vi "autoDrive.vi"(4 "Distance":dbl) -> (0 "right speed":dbl, 1 "left speed":dbl, 2 "finished?":bool)   [LabVIEW 2013]
doc: "Will drive the robot at a specified speed for a specified distance. Pretty simple."
uses:
  typedefs/fg_typedef.ctl
  typedefs/State Machine/subStates.ctl
  <vilib>/addons/control/pid/NI_PID_pid.lvlib
  <vilib>/addons/control/pid/pid.llb/PID (DBL).vi
panel:
  out "right desired rate":dbl
  out "left desired rate":dbl
  out "leftDistance":dbl
  out "rightDistance":dbl
  out "leftRate":dbl
  out "rightRate":dbl
  # "Encoder Data"
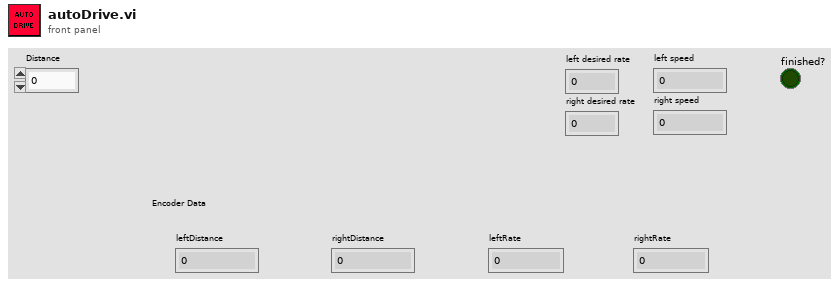
[diagram p1: front panel]
types:
  T1 = typedef "subStates.ctl" = enum16{"null", "wait", "driver control", "auto", "manual override", "hold position", "rotate", "pickup", "pass", "recover pass", "load", "goto shoot", "shoot high goal", "shoot low goal", "cancel arm", "cancel shooter", "end", "test"}
  T2 = typedef "fg_typedef.ctl" = enum16{"Get", "Set"}
  T3 = typedef "WPI_EncoderDevRef.ctl" = cluster{"DevStatus":errorcluster, "EncoderIndex":T4, "CounterIndex":T5, "DistancePerCount":dbl, "Decoding Type":T6}
  T4 = typedef "FPGA_EncoderIdx.ctl" = enum8{"Enc 0", "Enc 1", "Enc 2", "Enc 3", "Invalid"}
  T5 = typedef "FPGA_CounterCtrSystemIndex.ctl" = enum8{"Ctr 0", "Ctr 1", "Ctr 2", "Ctr 3", "Ctr 4", "Ctr 5", "Ctr 6", "Ctr 7", "Invalid"}
  T6 = typedef "WPI_EncoderType.ctl" = enum16{"1x", "2x", "4x"}
  T7 = cluster{"proportional gain (Kc)":dbl, "integral time (Ti, min)":dbl, "derivative time (Td, min)":dbl}
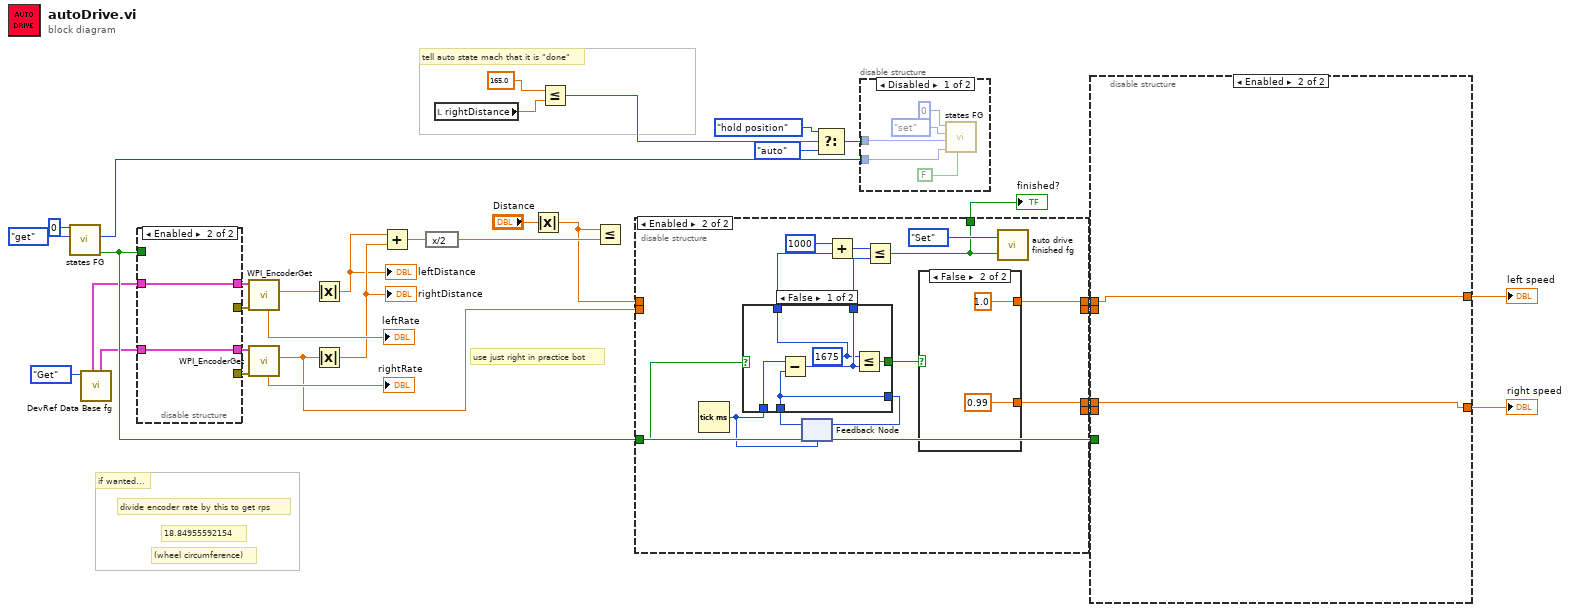
[diagram p0: block diagram]
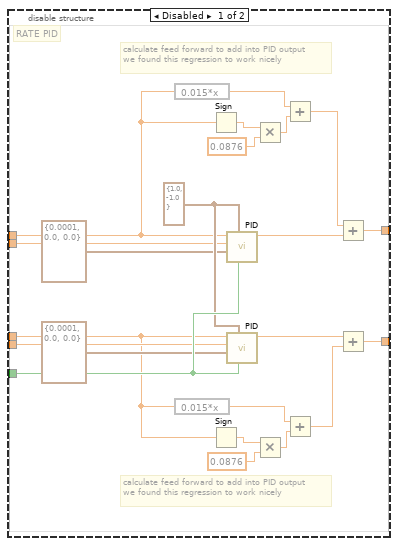
[diagram p3: hidden frame]
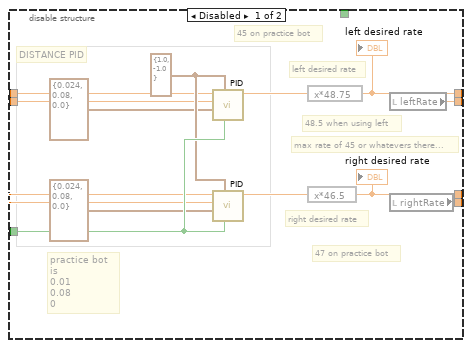
[diagram p4: hidden frame]
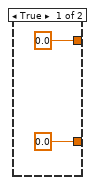
[diagram p5: hidden frame]
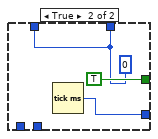
[diagram p6: hidden frame]
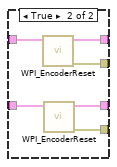
[diagram p8: hidden frame]
diagram:
  # "if wanted..."
  # "tell auto state mach that it is \"done\""
  # "use just right in practice bot"
  # "(wheel circumference)"
  # "divide encoder rate by this to get rps"
  # "18.84955592154"
  n1 = call "states FG.vi"("menu (get)"=enum16{"set", "get"}."get", "Loop ID"=0) -> ("first call?"=w34:bool, "state # out"=w26:i32)  [unwired: 6 in, 2 out]
  n2 = call "DevRef Data Base fg.vi"("Menu"=fg_typedef."Get") -> ("right drive encoder"=w23:T3, "left drive encoder"=w24:T3)  [unwired: 2 in, 7 out]
  n3 = disable-structure shown="Enabled" {
    disable-tunnel: w24 -> [w41 w51]
    disable-tunnel: w23 -> [w40 w50]
    disable-tunnel: [w39 _] -> w32
    disable-tunnel: [w38 w51] -> w31
    disable-tunnel: [w37 w50] -> w30
    disable-tunnel: [w36 _] -> w29
    disable-tunnel: w34 -> [w35 _]
    frame Disabled {
      n4 = case shown="False" w35 {
        tunnel: w41 -> [w43 w48]
        tunnel: w40 -> [w42 w46]
        tunnel: [_ w49] -> w39
        tunnel: [w43 w47] -> w38
        tunnel: [w42 w45] -> w37
        tunnel: [_ w44] -> w36
        frame False {
        }
        frame True {
          n5 = call <vilib>:"WPI_EncoderReset.vi"("EncoderDevRef"=w48) -> ("error out"=w49:errorcluster, "EncoderDevRef"=w47:T3)  [unwired: 9 in]
          n6 = call <vilib>:"WPI_EncoderReset.vi"("EncoderDevRef"=w46) -> ("error out"=w44:errorcluster, "EncoderDevRef"=w45:T3)  [unwired: 9 in]
        }
      }
    }
    frame Enabled {
    }
  }
  n7 = call <vilib>:"WPI_EncoderGet.vi"("error in (no error)"=w32, "EncoderDevRef"=w31) -> ("Distance"=w4:dbl, "Rate"=→"leftRate":dbl)  [unwired: 4 in, 4 out]
  n8 = call <vilib>:"WPI_EncoderGet.vi"("error in (no error)"=w29, "EncoderDevRef"=w30) -> ("Distance"=w3:dbl, "Rate"=→"rightRate":dbl)  [unwired: 4 in, 4 out]
  n9 = Absolute Value(x=w4) -> (abs(x)=w11:dbl)
  "leftDistance" <- w11
  n10 = Absolute Value(x=w3) -> (abs(x)=w14:dbl)
  "rightDistance" <- w14
  n11 = Add(x=w11, y=w14) -> (x+y=w13:dbl)
  n12 = expression code="x/2"(w13) -> (w12:dbl)
  n13 = local read "rightDistance"() -> (w8:dbl)
  n14 = Absolute Value(x="Distance") -> (abs(x)=w7:dbl)
  n15 = Less Or Equal?(x=165.0, y=w8) -> (x <= y?=w2:bool)
  n16 = Less Or Equal?(x=w7, y=w12) -> ()  [unwired: 1 out]
  n17 = disable-structure shown="Enabled" {
    disable-tunnel: w34 -> [w63 w71]
    disable-tunnel: [w58 _] -> w18
    disable-tunnel: [w57 _] -> w17
    disable-tunnel: [w56 w76] -> w16
    disable-tunnel: [w54 w75] -> w15
    disable-tunnel: w7 -> [w53 _]
    disable-tunnel: w3 -> [w52 _]
    disable-tunnel: [_ w67] -> w1
    frame Disabled {
      w60 = cluster{"output high":dbl, "output low":dbl} {"output high"=1.0, "output low"=-1.0} ("output range")
      # "DISTANCE PID"
      # "48.5 when using left"
      # "practice bot is \n0.01\n0.08\n0"
      # "45 on practice bot"
      # "47 on practice bot"
      # "max rate of 45 or whatevers there..."
      # "left desired rate"
      # "right desired rate"
      n18 = call-poly <vilib>:"PID.vi"("reinitialize? (F)"=w63, "output range"=w60, "PID gains"=T7 {"proportional gain (Kc)"=0.024, "integral time (Ti, min)"=0.08, "derivative time (Td, min)"=0.0} ("Left Distance PID gains"), "process variable"=w52, "setpoint"=w53) -> ("output"=w62:dbl)  [unwired: 5 in, 1 out]
      n19 = call-poly <vilib>:"PID.vi"("reinitialize? (F)"=w63, "output range"=w60, "PID gains"=T7 {"proportional gain (Kc)"=0.024, "integral time (Ti, min)"=0.08, "derivative time (Td, min)"=0.0} ("Right Distance PID gains"), "process variable"=w52, "setpoint"=w53) -> ("output"=w61:dbl)  [unwired: 5 in, 1 out]
      n20 = expression code="x*48.75"(w62) -> (w56:dbl)
      "left desired rate" <- w56
      n21 = expression code="x*46.5"(w61) -> (w54:dbl)
      "right desired rate" <- w54
      n22 = local read "leftRate"() -> (w58:dbl)
      n23 = local read "rightRate"() -> (w57:dbl)
    }
    frame Enabled {
      n24 = Tick Count (ms)() -> (millisecond timer value=w72:u32)
      n25 = feedback #1(w72) -> (w74:u32)
      n26 = case shown="False" w71 {
        tunnel: w72 -> [w85 _]
        tunnel: [w83 w88] -> w73
        tunnel: w74 -> [w83 _]
        tunnel: [w84 TRUE] -> w70
        tunnel: [w82 w86] -> w68
        tunnel: [w81 w86] -> w65
        frame False {
          w81 = u32 1675 ("x")
          n27 = Subtract(x=w85, y=w83) -> (x-y=w82:u32)
          n28 = Less Or Equal?(x=w81, y=w82) -> (x <= y?=w84:bool)
        }
        frame True {
          w86 = u32 0
          n29 = Tick Count (ms)() -> (millisecond timer value=w88:u32)
        }
      }
      n30 = feedback-in #1(w73) -> ()
      n31 = Add(x=u32 1000, y=w65) -> (x+y=w66:u32)
      n32 = Less Or Equal?(x=w66, y=w68) -> (x <= y?=w67:bool)
      n33 = case shown="False" w70 {
        tunnel: [0.0 ("output") 1.0 ("output")] -> w76
        tunnel: [0.0 ("output") 0.99 ("output")] -> w75
        frame True {
        }
        frame False {
        }
      }
      n34 = call "auto drive finished fg.vi"("Done?"=w67, "Menu"=fg_typedef."Set") -> ()  [unwired: 1 out]
    }
  }
  "finished?" <- w1
  n35 = Select(t=subStates."hold position" ("subState in"), s=w2, f=subStates."auto") -> (s? t:f=w9:T1)
  n36 = disable-structure shown="Disabled" {
    disable-tunnel: w26 -> [w93 _]
    disable-tunnel: w9 -> [w90 _]
    frame Disabled {
      n37 = call "states FG.vi"("exit in"=FALSE, "state # in"=w93, "subState in"=w90, "menu (get)"=enum16{"set", "get"}."set", "Loop ID"=0) -> ()  [unwired: 3 in, 4 out]
    }
    frame Enabled {
    }
  }
  n38 = disable-structure shown="Enabled" {
    disable-tunnel: w34 -> [w115 _]
    disable-tunnel: [w111 w117] -> w22
    disable-tunnel: [w110 w116] -> w21
    disable-tunnel: w18 -> [w108 _]
    disable-tunnel: w17 -> [w107 _]
    disable-tunnel: w16 -> [w100 w117]
    disable-tunnel: w15 -> [w94 w116]
    frame Disabled {
      w109 = cluster{"output high":dbl, "output low":dbl} {"output high"=1.0, "output low"=-1.0} ("output range")
      # "RATE PID"
      # "calculate feed forward to add into PID output\nwe found this regression to work nicely"
      # "calculate feed forward to add into PID output\nwe found this regression to work nicely"
      n39 = expression code="0.015*x"(w100) -> (w103:dbl)
      n40 = expression code="0.015*x"(w94) -> (w99:dbl)
      n41 = Sign(1:w100) -> (0:w106:dbl)
      n42 = Sign(1:w94) -> (0:w96:dbl)
      n43 = call-poly <vilib>:"PID.vi"("reinitialize? (F)"=w115, "output range"=w109, "PID gains"=T7 {"proportional gain (Kc)"=0.0001, "integral time (Ti, min)"=0.0, "derivative time (Td, min)"=0.0} ("Left Rate PID gains"), "process variable"=w108, "setpoint"=w100) -> ("output"=w102:dbl)  [unwired: 5 in, 1 out]
      n44 = call-poly <vilib>:"PID.vi"("reinitialize? (F)"=w115, "output range"=w109, "PID gains"=T7 {"proportional gain (Kc)"=0.0001, "integral time (Ti, min)"=0.0, "derivative time (Td, min)"=0.0} ("Right Rate PID gains"), "process variable"=w107, "setpoint"=w94) -> ("output"=w112:dbl)  [unwired: 5 in, 1 out]
      n45 = Multiply(x=w106, y=0.0876) -> (x*y=w104:dbl)
      n46 = Multiply(x=w96, y=0.0876) -> (x*y=w98:dbl)
      n47 = Add(x=w103, y=w104) -> (x+y=w101:dbl)
      n48 = Add(x=w99, y=w98) -> (x+y=w114:dbl)
      n49 = Add(x=w101, y=w102) -> (x+y=w111:dbl)
      n50 = Add(x=w112, y=w114) -> (x+y=w110:dbl)
    }
    frame Enabled {
    }
  }
  "left speed" <- w22
  "right speed" <- w21
